vi "Digitizer Synch.vi"(8 "error in":errorcluster, 11 "Channel Parameters In":T1={"Channel Name"="0", "Number of Records"=0, "Reference Position"=0.0, "Minimum Record Length"=0, "Minimum Sample Rate"=0.0, "Maximum Input Frequency"=0.0, "Enforce Realtime"=FALSE, "Vertical Coupling"=enum."AC", "Probe Attenuation"=0.0, "Vertical Range (V)"=0.0, "Vertical Offset"=0.0, "Trigger Level"=0.0, "Trigger Type"=enum."Edge", "Trigger Source"=enum."Immediate", "Trigger Slope"=enum."Positive", "Digitizer 1 Used?"=FALSE, "Digitizer 1 Channels"="", "Digitizer 1 Reference"="", "Digitizer 1 Gain Multiplier"=nan, "Digitizer 2 Used?"=FALSE, "Digitizer 2 Channels"="", "Digitizer 2 Reference"="", "Session References"=[]}) -> (0 "error out":errorcluster, 3 "Channel Parameters Out":T1={"Channel Name"="", "Number of Records"=0, "Reference Position"=0.0, "Minimum Record Length"=0, "Minimum Sample Rate"=0.0, "Maximum Input Frequency"=0.0, "Enforce Realtime"=FALSE, "Vertical Coupling"=enum."AC", "Probe Attenuation"=0.0, "Vertical Range (V)"=0.0, "Vertical Offset"=0.0, "Trigger Level"=0.0, "Trigger Type"=enum."Edge", "Trigger Source"=enum."Immediate", "Trigger Slope"=enum."Positive", "Digitizer 1 Used?"=FALSE, "Digitizer 1 Channels"="", "Digitizer 1 Reference"="", "Digitizer 1 Gain Multiplier"=nan, "Digitizer 2 Used?"=FALSE, "Digitizer 2 Channels"="", "Digitizer 2 Reference"="", "Session References"=[]})   [LabVIEW 2010]
uses:
  Typedef-Channel Parameters.ctl
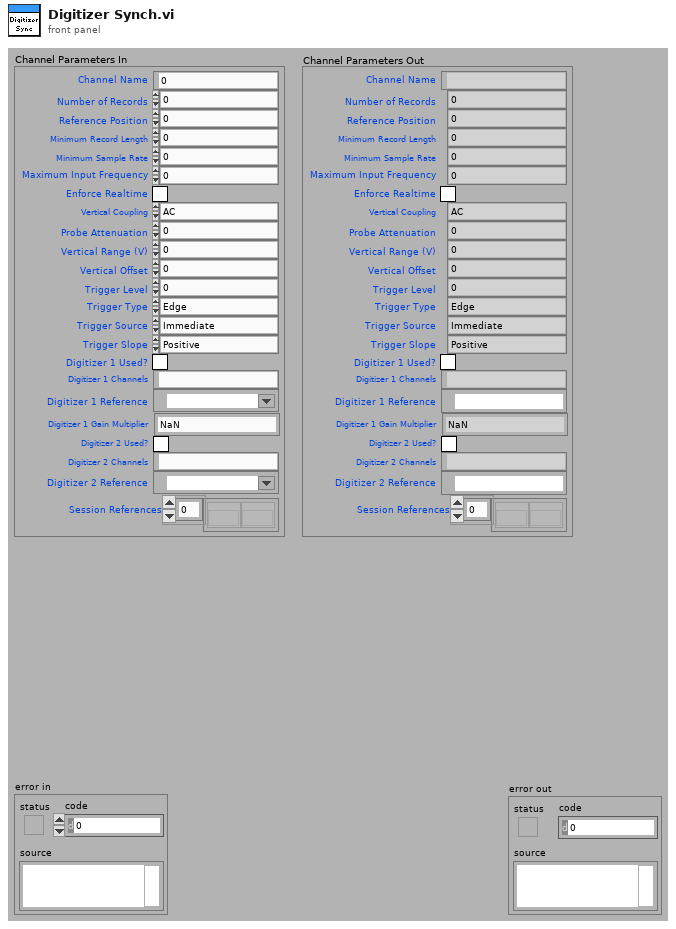
[diagram p1: front panel]
types:
  T1 = typedef "Typedef-Channel Parameters.ctl" = cluster{"Channel Name":string, "Number of Records":i32, "Reference Position":dbl, "Minimum Record Length":i32, "Minimum Sample Rate":dbl, "Maximum Input Frequency":dbl, "Enforce Realtime":bool, "Vertical Coupling":enum16{"AC", "DC", "Ground"}, "Probe Attenuation":dbl, "Vertical Range (V)":dbl, "Vertical Offset":dbl, "Trigger Level":dbl, "Trigger Type":enum16{"Edge", "Digital", "Immediate"}, "Trigger Source":enum16{"Immediate", "Channel 0", "Channel 1", "Channel 2", "Channel 3", "Channel 4", "Channel 5", "Channel 6", "Channel 7", "Extermal TRIG", "Software Trigger", "RTSI 0", "RTSI 1", "RTSI 2", "RTSI 3", "RTSI 4", "RTSI 5", "RTSI 6", "PF 0", "PF 1", "PF 2", "PXI Star Trigger"}, "Trigger Slope":enum16{"Positive", "Negative"}, "Digitizer 1 Used?":bool, "Digitizer 1 Channels":string, "Digitizer 1 Reference":refnum<k15>, "Digitizer 1 Gain Multiplier":dbl, "Digitizer 2 Used?":bool, "Digitizer 2 Channels":string, "Digitizer 2 Reference":refnum<k15>, "Session References":refnum<k20>[]}
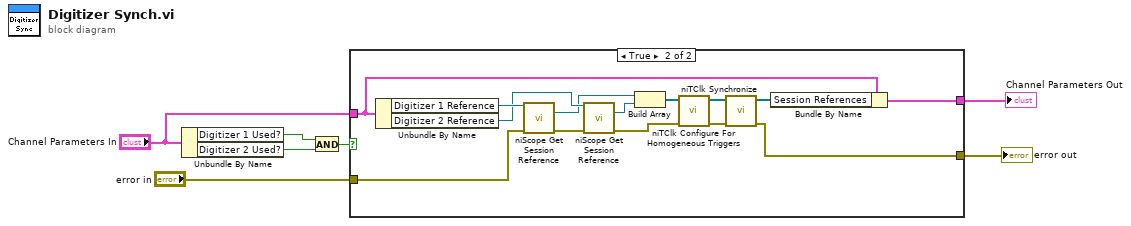
[diagram p0: block diagram]
diagram:
  n1 = Unbundle By Name("Channel Parameters In") -> ("Digitizer 1 Used?"=w7:bool, "Digitizer 2 Used?"=w6:bool)
  n2 = And(x=w7, y=w6) -> (x .and. y?=w5:bool)
  n3 = case shown="True" w5 {
    tunnel: "Channel Parameters In" -> [w8 w12]
    tunnel: "error in" -> [w9 w14]
    tunnel: [w9 w13] -> w2
    tunnel: [w8 w10] -> w1
    frame False {
    }
    frame True {
      n4 = Unbundle By Name(w12) -> ("Digitizer 1 Reference"=w21:refnum<k15>, "Digitizer 2 Reference"=w19:refnum<k15>)
      n5 = call <instrlib>:"niScope Get Session Reference.vi"("instrument handle"=w21, "error in"=w14) -> ("session reference"=w18:refnum<k20>, "error out"=w20:errorcluster)  [unwired: 11 in, 1 out]
      n6 = call <instrlib>:"niScope Get Session Reference.vi"("instrument handle"=w19, "error in"=w20) -> ("session reference"=w17:refnum<k20>, "error out"=w22:errorcluster)  [unwired: 11 in, 1 out]
      n7 = Build Array(w18, w17) -> (w16:refnum<k20>[])
      n8 = call <instrlib>:"niTClk Configure For Homogeneous Triggers.vi"("error in (no error)"=w22, "sessions"=w16) -> ("error out"=w23:errorcluster, "sessions out"=w15:refnum<k20>[])  [unwired: 8 in]
      n9 = call <instrlib>:"niTClk Synchronize.vi"("error in (no error)"=w23, "sessions"=w15) -> ("error out"=w13:errorcluster, "sessions out"=w11:refnum<k20>[])  [unwired: 8 in]
      n10 = Bundle By Name(cluster=w12, "Session References"=w11) -> (w10:T1)
    }
  }
  "error out" <- w2
  "Channel Parameters Out" <- w1
